vi "正面处理test.vi"(7 "error in":errorcluster) -> (27 "error out":errorcluster)   [LabVIEW 2015]
uses:
  <vilib>/vision/Measure.llb/Edge Options.ctl
  <vilib>/vision/Measure.llb/Edge Polarity.ctl
  <vilib>/vision/Contour.llb/IMAQ Connect Range Setting.ctl
  <vilib>/vision/Contour.llb/IMAQ Contour Curve Extraction.ctl
  <vilib>/vision/Pattern Matching.llb/IMAQ Match Range Setting.ctl
  <vilib>/vision/NI_Vision_Development_Module.lvlib
panel:
  in  "ROI Descriptor":T1={"Global Rectangle"=[874, 1081, 1644, 1850], "Contours"=[{"ID"=enum."External", "Type"=7, "Coordinates"=[1258, 1465, 71, 384, 0, 0]}]} {"Contours"."Type" items=["No Selection", "Point", "Line", "Rectangle", "Oval", "Polygon", "Freehand Region", "Annulus", "Unused2", "Unused3", "Broken Line", "Freehand Line", "Rotated Rectangle"]}
  out "Fitted Circle":T2
  out "ROI Descriptor out 2":T3 {"Contours"."Type" items=["No Selection", "Point", "Line", "Rectangle", "Oval", "Polygon", "Freehand Region", "Annulus", "Unused2", "Unused3", "Broken Line", "Freehand Line", "Rotated Rectangle"]}
  out "ROI Descriptor out":T3 {"Contours"."Type" items=["No Selection", "Point", "Line", "Rectangle", "Oval", "Polygon", "Freehand Region", "Annulus", "Unused2", "Unused3", "Broken Line", "Freehand Line", "Rotated Rectangle"]}
  in  "Options":T6={"Search  Direction"=1, "Edge Options"={"Edge Polarity"=0, "Kernel Size"=3, "Width"=3, "Minimum Edge Strength"=178.0, "Interpolation Type"=enum."Bilinear Fixed", "Data Processing Method"=enum."Average"}, "Show Search Area"=TRUE, "Show Search Lines"=TRUE, "Show Edges Found"=TRUE, "Show Result"=TRUE, "Search Area Color"=65280, "Search Lines Color"=255, "Edge Locations Color"=16776960, "Result Color"=16711680, "Overlay Group Name"=""} {"Search  Direction" items=["Outside to Inside", "Inside to Outside"]; "Edge Options"."Edge Polarity" items=["All Edges", "Rising Edges", "Falling Edges"]; "Edge Options"."Minimum Edge Strength" format="%.2f"; "Edge Options"."Width" step=2; "Edge Options"."Kernel Size" step=2}
  out "Annulus":T7 {"End Angle" min=-90.0 max=90.0 step=1.0 format="%.2f"; "Start Angle" min=-90.0 max=90.0 step=1.0 format="%.2f"; "Center X" scale=0.0..1024.0}
  out "Image Out":T8(plugin-control)
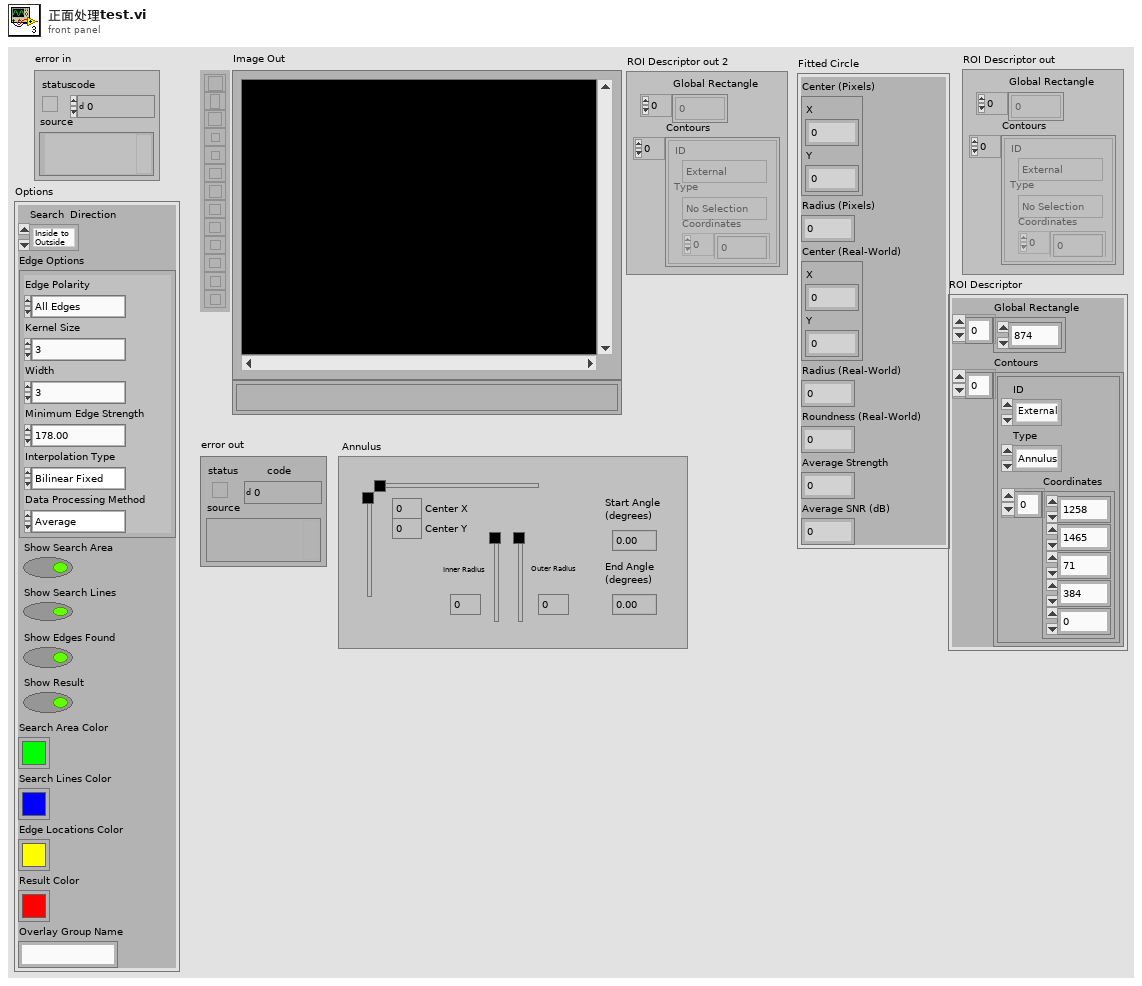
[diagram p1: front panel]
types:
  T1 = cluster{"Global Rectangle":i32[], "Contours":cluster{"ID":enum32{"External", "Internal"}, "Type":u32, "Coordinates":i32[]}[]}
  T2 = cluster{"Center (Pixels)":cluster{"X":sgl, "Y":sgl}, "Radius (Pixels)":dbl, "Center (Real-World)":cluster{"X":sgl, "Y":sgl}, "Radius (Real-World)":dbl, "Roundness (Real-World)":dbl, "Average Strength":dbl, "Average SNR (dB)":dbl}
  T3 = typedef "ROI Descriptor" = cluster{"Global Rectangle":i32[], "Contours":cluster{"ID":enum32{"External", "Internal"}, "Type":u32, "Coordinates":i32[]}[]}
  T4 = typedef "Edge Options.ctl" = cluster{"Edge Polarity":T5, "Kernel Size":u32, "Width":u32, "Minimum Edge Strength":sgl, "Interpolation Type":enum32{"Zero Order", "Bilinear", "Quadratic", "Cubic", "Bilinear Fixed"}, "Data Processing Method":enum32{"Average", "Median"}}
  T5 = typedef "Edge Polarity.ctl" = u32
  T6 = cluster{"Search  Direction":u32, "Edge Options":T4, "Show Search Area":bool, "Show Search Lines":bool, "Show Edges Found":bool, "Show Result":bool, "Search Area Color":u32, "Search Lines Color":u32, "Edge Locations Color":u32, "Result Color":u32, "Overlay Group Name":string}
  T7 = typedef "IMAQ Circle" = cluster{"Center X":i32, "Center Y":i32, "Inner Radius":i32, "Outer Radius":i32, "Start Angle":dbl, "End Angle":dbl}
  T8 = typedef "IMAQ Image.ctl" = refnum<image>
  T9 = enum16{"Horizontal Motion", "Vertical Motion", "Horizontal and Vertical Motion", "Horizontal, Vertical and Angular Motion"}
  T10 = cluster{"Rotation":bool, "Scale":bool, "Occlusion":bool}
  T11 = typedef "IMAQ Match Range Setting.ctl" = cluster{"Match Constraints":u32, "Min":dbl, "Max":dbl}
  T12 = cluster{"Setup Data Item":u16, "Item Value":dbl}[]
  T13 = typedef "IMAQ Contour Curve Extraction.ctl" = cluster{"Extraction Mode":u32, "Edge Threshold":i32, "Edge Filter Size":u32, "Min Length":i32, "Search Step Size":i32, "Max Endpoint Gap":i32, "Subpixel":bool}
  T14 = typedef "IMAQ Connect Range Setting.ctl" = cluster{"Match Constraints":u32, "Min":dbl, "Max":dbl}
  T15 = enum16{"Closest To Search Start", "Maximum Length", "Strongest Mean Gradient Change"}
  T16 = enum16{"Rect Left To Right", "Rect Right To Left", "Rect Top To Bottom", "Rect Bottom To Top", "Annulus Inner To Outer", "Annulus Outer To Inner", "Annulus Start Angle To End Angle", "Annulus End Angle To Start Angle"}
  T17 = cluster{"Overlay?":bool, "Color":u32, "Width":u32, "Maintain Width?":bool}
  T18 = cluster{"Origin":cluster{"X":sgl, "Y":sgl}, "Angle (deg)":sgl, "Axis Reference":u32}
  T19 = enum16{"Reset", "Update Coordinate System", "Get Coordinate System"}
  T20 = cluster{"Process":enum16{"Get First Edge", "Get First + Last Edge", "Get All Edges", "Get Best Edge"}, "Step Size":i32, "Max Pixel Radius":i32}
  T21 = cluster{"Measurement Parameter":i32, "Range Lower Value":dbl, "Range Upper Value":dbl, "Range":bool, "Measurement Type":bool}[]
  T22 = enum32{"AutoM", "Close", "Dilate", "Erode", "Gradient", "Gradient out", "Gradient in", "Hit miss", "Open", "PClose", "POpen", "Thick", "Thin"}
  T23 = typedef "Image Type" = u32
  T24 = cluster{"histogram":u32[], "Minimal Value":sgl, "Maximal Value":sgl, "Starting Value":sgl, "Interval Width":sgl, "Mean Value":sgl, "Standard  Variation":sgl, "Area (pixels)":i32}
  T25 = typedef "IMAQ Coordinate System" = cluster{"Reference System":cluster{"Origin":cluster{"X":sgl, "Y":sgl}, "Angle (deg)":sgl, "Axis Reference":u32}, "Measurement System":cluster{"Origin":cluster{"X":sgl, "Y":sgl}, "Angle (deg)":sgl, "Axis Reference":u32}}
  T26 = cluster{"Left":i32, "Top":i32, "Right":i32, "Bottom":i32}
  T27 = cluster{"Target Point":cluster{"X":dbl, "Y":dbl}, "Template Point":cluster{"X":dbl, "Y":dbl}, "Distance":dbl}[]
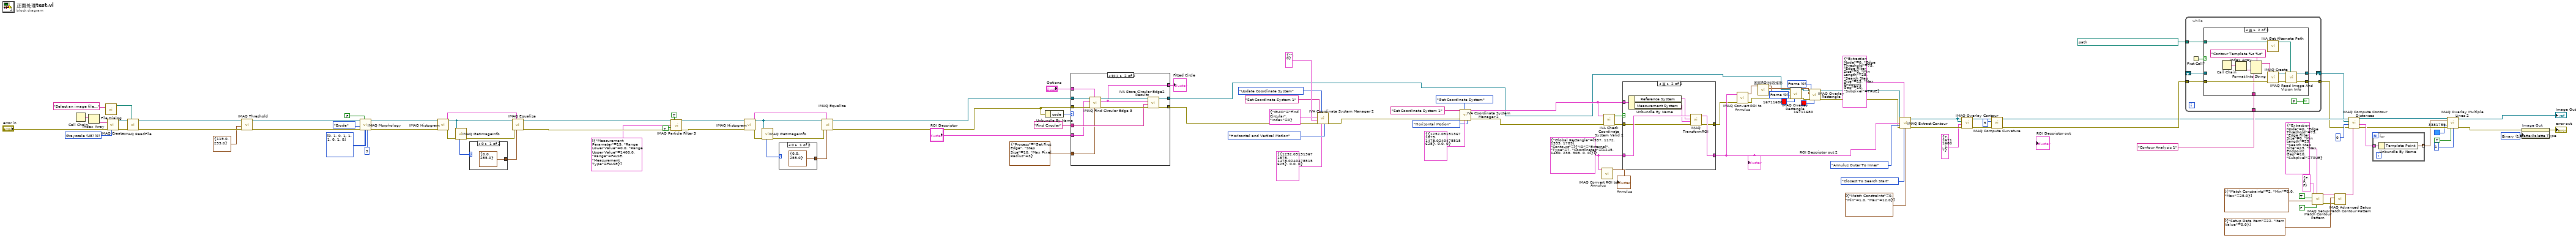
[diagram p0: block diagram]
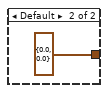
[diagram p5: hidden frame]
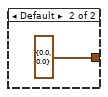
[diagram p6: hidden frame]
diagram:
  w8 = u32 0 items=["Frame", "Fill", "Highlight"] ("Drawing Mode (Frame)")
  w11 = u32 0 items=["Frame", "Fill", "Highlight"] ("Drawing Mode (Frame)")
  w20 = u32 1 items=["Grayscale", "Binary", "Gradient", "Rainbow", "Temperature", "User Defined", "Binary 16 Bit", "Gradient 16 Bit", "Rainbow 16 Bit", "Temperature 16 Bit", "User Defined 16 Bit"] ("Palette Type")
  w19 = T1 {"Global Rectangle"=[937, 1172, 1555, 1789], "Contours"=[{"ID"=enum."External", "Type"=7, "Coordinates"=[1245, 1480, 238, 308, 0, 0]}]} ("ROI Descriptor")
  w106 = T23 0 items=["Grayscale (U8)", "Grayscale (I16)", "Grayscale (SGL)", "Complex (CSG)", "RGB (U32)", "HSL (U32)", "RGB (U64)", "Grayscale (U16)"] ("Image Type")
  n1 = Call Chain() -> (call chain=w110:string[])
  n2 = Index Array(array=w110) -> (element=w109:string)  [unwired: 1 in]
  n3 = call "File Dialog"("prompt"="Select an image file...") -> ("selected path"=w107:path)  [unwired: 6 in, 8 out]
  n4 = call "IMAQ Create"("Image Name"=w109, "Image Type"=w106, "error in (no error)"="error in") -> ("New Image"=w113:T8, "error out"=w112:errorcluster)  [unwired: 1 in, 1 out]
  n5 = call "IMAQ ReadFile"("File Path"=w107, "error in (no error)"=w112, "Image"=w113) -> ("error out"=w114:errorcluster, "Image Out"=w104:T8)  [unwired: 2 in, 5 out]
  n6 = call "IMAQ Threshold"("error in (no error)"=w114, "Range"=cluster{"Lower value":sgl, "Upper value":sgl} {"Lower value"=119.0, "Upper value"=255.0}, "Image Src"=w104) -> ("error out"=w103:errorcluster, "Image Dst Out"=w98:T8)  [unwired: 3 in, 4 out]
  n7 = call "IMAQ Morphology"("Number of iterations (1)"=3, "Structuring Element"=i32[][] [[0, 1, 0], [1, 1, 1], [0, 1, 0]], "Square/Hexa (Square)"=FALSE, "error in (no error)"=w103, "Operation"=T22."Erode", "Image Src"=w98) -> ("error out"=w97:errorcluster, "Image Dst Out"=w93:T8)  [unwired: 1 in, 3 out]
  n8 = call "IMAQ Histogram"("error in (no error)"=w97, "Image"=w93) -> ("error out"=w92:errorcluster, "Histogram Report"=w95:T24)  [unwired: 3 in, 5 out]
  n9 = call "IMAQ GetImageInfo"("error in (no error)"=w92, "Image"=w93) -> ("error out"=w91:errorcluster, "Image Type"=w94:T23)  [unwired: 8 out]
  n10 = case "条件结构" shown="0" w94 {
    tunnel: [cluster{"Minimum":sgl, "Maximum":sgl} {"Minimum"=0.0, "Maximum"=255.0} ("Range") cluster{"Minimum":sgl, "Maximum":sgl} {"Minimum"=0.0, "Maximum"=0.0} ("Range")] -> w90
    frame 0 {
    }
    frame Default {
    }
  }
  n11 = call "IMAQ Equalize"("Range"=w90, "Histogram Report"=w95, "error in (no error)"=w91, "Image Src"=w93) -> ("error out"=w96:errorcluster, "Image Dst Out"=w86:T8)  [unwired: 2 in, 4 out]
  n12 = call "IMAQ Particle Filter 3"("Image Src"=w86, "Connectivity 4/8 (8)"=TRUE, "Selection Values"=T21 [{"Measurement Parameter"=19, "Range Lower Value"=0.0, "Range Upper Value"=1400.0, "Range"=FALSE, "Measurement Type"=FALSE}], "Keep/Remove Particles (F)"=TRUE ("Keep/Remove Particles"), "error in (no error)"=w96) -> ("Image Dst Out"=w81:T8, "error out"=w87:errorcluster)  [unwired: 4 in, 5 out]
  n13 = call "IMAQ Histogram"("error in (no error)"=w87, "Image"=w81) -> ("error out"=w80:errorcluster, "Histogram Report"=w83:T24)  [unwired: 3 in, 5 out]
  n14 = call "IMAQ GetImageInfo"("error in (no error)"=w80, "Image"=w81) -> ("error out"=w79:errorcluster, "Image Type"=w82:T23)  [unwired: 8 out]
  n15 = case "条件结构" shown="0" w82 {
    tunnel: [cluster{"Minimum":sgl, "Maximum":sgl} {"Minimum"=0.0, "Maximum"=255.0} ("Range") cluster{"Minimum":sgl, "Maximum":sgl} {"Minimum"=0.0, "Maximum"=0.0} ("Range")] -> w78
    frame 0 {
    }
    frame Default {
    }
  }
  n16 = call "IMAQ Equalize"("Range"=w78, "Histogram Report"=w83, "error in (no error)"=w79, "Image Src"=w81) -> ("error out"=w84:errorcluster, "Image Dst Out"=w77:T8)  [unwired: 2 in, 4 out]
  n17 = Unbundle By Name(w84) -> ("code"=w73:i32)
  n18 = case "条件结构" shown="默认" w73 {
    tunnel: "Options" -> [_ w120]
    tunnel: w77 -> [w119 w130]
    tunnel: w84 -> [_ w129]
    tunnel: [_ w127] -> w76
    tunnel: [w119 w125] -> w5
    tunnel: "Find Circular" ("Step Name") -> [_ w124]
    tunnel: "ROI Descriptor" -> [_ w123]
    tunnel: T20 {"Process"=enum."Get First Edge", "Step Size"=10, "Max Pixel Radius"=3} ("Circle Fit Options") -> [_ w122]
    tunnel: [_ w121] -> w2
    frame -1074396199, -1074396198 {
      # "Discard Coordinate System Error"
    }
    frame Default {
      n19 = call "IMAQ Find Circular Edge 3"("Circle Fit Options"=w122, "Options"=w120, "error in (no error)"=w129, "ROI Descriptor"=w123, "Image"=w130) -> ("error out"=w128:errorcluster, "Fitted Circle"=w121:T2, "Image Out"=w126:T8)  [unwired: 2 in, 2 out]
      n20 = call <vilib>:"IVA Store Circular Edge2 Results.vi"("error in (no error)"=w128, "Step Name"=w124, "Fitted Circle"=w121, "Image in"=w126) -> ("error out"=w127:errorcluster, "Image dup"=w125:T8)  [unwired: 2 in, 4 out]
    }
  }
  "Fitted Circle" <- w2
  n21 = call <vilib>:"IVA Coordinate System Manager 2.vi"("Mode"=T9."Horizontal and Vertical Motion", "Reference System"=T18 {"Origin"={"X"=1252.0515, "Y"=1478.024}, "Angle (deg)"=0.0, "Axis Reference"=0}, "Function"=T19."Update Coordinate System", "error in (no error)"=w76, "Angle ID"=cluster{"GUID":string, "Index":i32} {"GUID"="", "Index"=0}, "Origin ID"=cluster{"GUID":string, "Index":i32} {"GUID"="Find Circular", "Index"=0}, "Coordinate System Name"="Set Coordinate System 1") -> ("error out"=w64:errorcluster)  [unwired: 4 out]
  n22 = call <vilib>:"IVA Coordinate System Manager 2.vi"("Mode"=T9."Horizontal Motion", "Reference System"=T18 {"Origin"={"X"=1252.0515, "Y"=1478.024}, "Angle (deg)"=0.0, "Axis Reference"=0}, "Function"=T19."Get Coordinate System", "error in (no error)"=w64, "Coordinate System Name"="Set Coordinate System 1") -> ("error out"=w61:errorcluster, "Coordinate System Out"=w59:T25)  [unwired: 2 in, 3 out]
  n23 = call "IMAQ Convert ROI to Annulus"("ROI Descriptor"=w19) -> ("Annulus"=→"Annulus":T7)  [unwired: 8 in, 1 out]
  n24 = call <vilib>:"IVA Check Coordinate System Valid 2.vi"("error in (no error)"=w61, "Coordinate System"=w59) -> ("error out"=w57:errorcluster, "Valid?"=w58:bool)  [unwired: 8 out]
  n25 = case "条件结构" shown="真" w58 {
    tunnel: w19 -> [w132 w139]
    tunnel: [w132 w136] -> w7
    tunnel: [w131 w135] -> w6
    tunnel: w59 -> [_ w134]
    tunnel: w57 -> [w131 w133]
    frame False {
    }
    frame True {
      n26 = Unbundle By Name(w134) -> ("Reference System"=w138:T18, "Measurement System"=w137:T18)
      n27 = call "IMAQ TransformROI"("error in (no error)"=w133, "New Reference"=w137, "Base Reference"=w138, "ROI Descriptor"=w139) -> ("error out"=w135:errorcluster, "ROI Descriptor out"=w136:T3)  [unwired: 6 out]
    }
  }
  "ROI Descriptor out 2" <- w7
  n28 = call "IMAQ Convert ROI to Annulus"("error in (no error)"=w6, "ROI Descriptor"=w7) -> ("error out"=w16:errorcluster, "Annulus"=w14:T7)  [unwired: 7 in]
  n29 = call "圆环ROI转双矩形.vi"("Annulus 2"=w14) -> ("内环"=w12:T26, "外环"=w13:T26)  [unwired: 9 in]
  n30 = call "IMAQ Overlay Rectangle"("Color"=u32 16711680, "error in (no error)"=w16, "Drawing Mode (Frame)"=w11, "Rectangle"=w13, "Image"=w5) -> ("error out"=w15:errorcluster, "Image Out"=w17:T8)  [unwired: 5 in]
  n31 = call "IMAQ Overlay Rectangle"("Color"=u32 16711680, "error in (no error)"=w15, "Drawing Mode (Frame)"=w8, "Rectangle"=w12, "Image"=w17) -> ("error out"=w3:errorcluster, "Image Out"=w4:T8)  [unwired: 5 in]
  n32 = call "IMAQ Extract Contour"("Source Image"=w4, "Curve Extraction"=T13 {"Extraction Mode"=0, "Edge Threshold"=75, "Edge Filter Size"=0, "Min Length"=25, "Search Step Size"=15, "Max Endpoint Gap"=10, "Subpixel"=TRUE}, "ROI Descriptor"=w7, "Search Direction"=T16."Annulus Outer To Inner", "error in (no error)"=w3, "Contour Selection"=T15."Closest To Search Start", "Curve Connection"=T14[] [{"Match Constraints"=0, "Min"=1.0, "Max"=12.0}]) -> ("Source Image Out"=w50:T8, "error out"=w56:errorcluster)  [unwired: 1 in, 6 out]
  n33 = call "IMAQ Overlay Contour"("error in (no error)"=w56, "Contour Points Settings"=T17 {"Overlay?"=TRUE, "Color"=16711680, "Width"=1, "Maintain Width?"=TRUE}, "Contour Image"=w50, "Image"=w50) -> ("error out"=w54:errorcluster, "Image Out"=w48:T8)  [unwired: 2 in, 4 out]
  n34 = call "IMAQ Compute Curvature"("error in (no error)"=w54, "Kernel Width"=u32 5, "Contour Image"=w48) -> ("error out"=w47:errorcluster, "Contour Image Out (dup)"=w42:T8)  [unwired: 1 in, 6 out]
  n35 = while "While循环" {
    tunnel: path "C:/Users/hedongpo/Desktop/吕亚/Temp3.png" ("Template File Path") -> [w147]
    tunnel: "Contour Analysis 1" ("Step Name") -> [w145]
    shift-right: [w143] -> w41
    shift-left: _ -> [w144]
    tunnel: w47 -> [w142]
    tunnel: [w141] -> w40
    stop <- FALSE continue-if-true
    n36 = First Call?() -> (First Call?: T/F=w146:bool)
    n37 = case "条件结构" shown="真" w146 {
      tunnel: [w149 w151] -> w143
      tunnel: w144 -> [w149 _]
      tunnel: [w148 w150] -> w141
      tunnel: w142 -> [w148 w156]
      tunnel: w147 -> [_ w161]
      tunnel: w145 -> [_ w152]
      frame False {
      }
      frame True {
        n38 = Call Chain() -> (call chain=w158:string[])
        n39 = Index Array(array=w158) -> (element=w157:string)  [unwired: 1 in]
        n40 = Format Into String(format string="Contour Template %s %s" ("Image Name"), w157, w152) -> (resulting string=w160:string)  [unwired: 2 in, 1 out]
        n41 = call <vilib>:"IVA Get Alternate Path.vi"("Path In"=w161) -> ("Path Out"=w153:path)  [unwired: 10 out]
        n42 = call "IMAQ Create"("Image Name"=w160, "error in (no error)"=w156) -> ("New Image"=w155:T8, "error out"=w154:errorcluster)  [unwired: 2 in, 1 out]
        n43 = call "IMAQ Read Image And Vision Info"("File Path"=w153, "error in (no error)"=w154, "Image"=w155) -> ("error out"=w150:errorcluster, "Image Out"=w151:T8)  [unwired: 1 in, 6 out]
      }
    }
  }
  n44 = call "IMAQ Setup Match Contour Pattern"("Use Learn Curve Extraction"=FALSE, "Curve Extraction"=T13 {"Extraction Mode"=0, "Edge Threshold"=75, "Edge Filter Size"=0, "Min Length"=25, "Search Step Size"=15, "Max Endpoint Gap"=10, "Subpixel"=TRUE} ("Curve Extraction 2"), "Range Settings"=T11[] [{"Match Constraints"=2, "Min"=0.0, "Max"=25.0}], "Subpixel Accuracy"=TRUE, "Match Mode"=T10 {"Rotation"=FALSE, "Scale"=FALSE, "Occlusion"=FALSE}) -> ("error out"=w23:errorcluster, "Match Contour Pattern Setup Data"=w27:string)  [unwired: 1 in, 4 out]
  n45 = call "IMAQ Advanced Setup Match Contour Pattern"("Match Contour Pattern Setup Data In"=w27, "Advanced Contour Match Options"=T12 [{"Setup Data Item"=22, "Item Value"=0.0}], "error in (no error)"=w23) -> ("Match Contour Pattern Setup Data Out"=w26:string)  [unwired: 7 out]
  n46 = call "IMAQ Compute Contour Distances"("Match Contour Pattern Setup Data"=w26, "error in (no error)"=w40, "Smoothing Kernel"=u32 0, "Template Contour Image"=w41, "Target Contour Image"=w42) -> ("error out"=w34:errorcluster, "Distances"=w36:T27, "Target Contour Image Out (dup)"=w35:T8)  [unwired: 4 out]
  n47 = for "For循环" {
    tunnel: w36 -> [w163] mode=indexing
    tunnel: [w162] -> w33 mode=indexing
    n48 = Unbundle By Name(w163) -> ("Template Point"=w162:cluster{"X":dbl, "Y":dbl})
  }
  n49 = call "IMAQ Overlay Multiple Lines 2"("Image"=w35, "Line End Points"=w33, "Color"=u32 3381759, "error in (no error)"=w34, "Maintain Width?"=TRUE, "Width"=u32 1) -> ("Image Out"=→"Image Out":T8, "error out"=w30:errorcluster)  [unwired: 2 in, 6 out]
  n50 = property on="Image Out" class="ImageControl"(error in=w30, "Palette:Palette Type"=w20) -> (error out=→"error out":errorcluster)  [unwired: 1 in, 1 out]
